vi "initHardwareList.vi"(8 "error in (no error)":errorcluster, 10 "HardwareList out":refnum<class "HWConfiguration.lvclass">, 11 "BECHWCBasic in":refnum<class "BECHWCBasic.lvclass">) -> (0 "error out":errorcluster, 3 "BECHWCBasic out":refnum<class "BECHWCBasic.lvclass">)   [LabVIEW 2011, in "Hardware.lvlib" / "HWControllers.lvlib" / "BECHWCBasic.lvclass"]
doc: "initialise hardware list."
uses:
  BECHWCBasic.lvclass
  HardwareConfiguration/HWConfiguration.lvclass
  BECHWCBasic.lvclass/BECHWCBasic.ctl
  HWController.lvclass
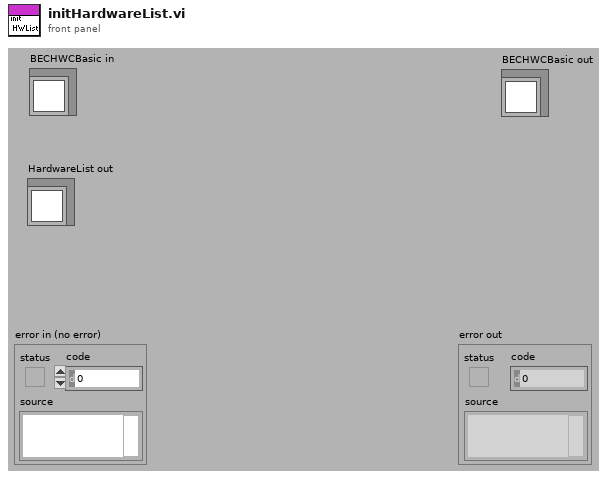
[diagram p1: front panel]
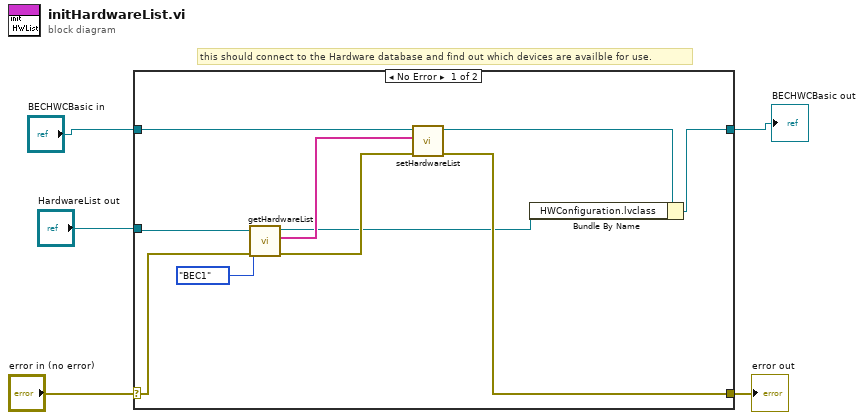
[diagram p0: block diagram]
diagram:
  # "this should connect to the Hardware database and find out which devices are availble for use."
  n1 = case shown="No Error" "error in (no error)" {
    selector: "error in (no error)" -> [w6 w17]
    tunnel: [w11 w17] -> w4
    tunnel: [w8 w16] -> w2
    tunnel: "BECHWCBasic in" -> [w14 w16]
    tunnel: "HardwareList out" -> [w7 _]
    frame No Error {
      n2 = call "getHardwareList.vi"("error in (no error)"=w6, "Enum"=enum16{"BEC1", "BEC2", "SingleAtom", "Testing"}."BEC1", "HWConfiguration in"=w7) -> ("error out"=w12:errorcluster, "HWList"=w13:string[], "HWConfiguration out"=w10:refnum<class "HWConfiguration.lvclass">)  [unwired: 6 in]
      n3 = call "setHardwareList.vi"("error in (no error)"=w12, "hardwareList"=w13, "HWController in"=w14) -> ("error out"=w11:errorcluster, "HWController out"=w9:refnum<class "BECHWCBasic.lvclass">)  [unwired: 7 in]
      n4 = Bundle By Name(cluster=w9, "HWConfiguration.lvclass"=w10) -> (w8:refnum<class "BECHWCBasic.lvclass">)
    }
    frame Error {
    }
  }
  "error out" <- w4
  "BECHWCBasic out" <- w2
